vi "Calculate Curvatures.vi"(8 "error in (no error)":errorcluster, 11 "EdgeDetectionProcessor in":refnum<class "EdgeDetectionProcessor.lvclass">) -> (0 "error out":errorcluster, 3 "EdgeDetectionProcessor out":refnum<class "EdgeDetectionProcessor.lvclass">)   [LabVIEW 2018, in "EdgeDetectionProcessor.lvclass"]
uses:
  EdgeDetectionProcessor.lvclass
  C:/Program Files/National Instruments/LabVIEW 2018/user.lib/Aaron/File IO/Video/Video Processor/Video Processor.lvclass
  private/Curvature Data STYP.ctl
  2471ccb5-288c-48cc-980c-5038d1df1be7.vi
  <vilib>/Analysis/5stat.llb/RMS (DBL).vi
  <vilib>/Analysis/baseanly.llb/Mean (DBL).vi
  2471ccb5-288c-48cc-980c-5038d1df1be7.vi/1ebe9616-e55e-4f0d-8ff4-2807f1f9a203.vi
  2471ccb5-288c-48cc-980c-5038d1df1be7.vi/377cf58b-8b4d-454a-95e9-e3c545549c0f.vi
  2471ccb5-288c-48cc-980c-5038d1df1be7.vi/c9f4e0f8-7816-4916-bc5d-49cbeb604e66.vi
  2471ccb5-288c-48cc-980c-5038d1df1be7.vi/08091d57-9891-4f86-b7e8-c83c60ad9e1e.vi
  2471ccb5-288c-48cc-980c-5038d1df1be7.vi/9f18ae6c-b72e-49ca-819e-288b80c2ac08.vi
  2471ccb5-288c-48cc-980c-5038d1df1be7.vi/60678d55-dfb7-4c78-a7ca-2aeac6e8a501.vi
  <vilib>/Analysis/2dsp.llb/Derivative x(t).vi
  2471ccb5-288c-48cc-980c-5038d1df1be7.vi/1ebe9616-e55e-4f0d-8ff4-2807f1f9a203.vi/a5d5fd81-05cf-4e8b-aa3e-5fb4ea73c4ff.vi
  2471ccb5-288c-48cc-980c-5038d1df1be7.vi/377cf58b-8b4d-454a-95e9-e3c545549c0f.vi/45177a7b-6163-4512-95a4-701ed642dc24.vi
  2471ccb5-288c-48cc-980c-5038d1df1be7.vi/08091d57-9891-4f86-b7e8-c83c60ad9e1e.vi/465288f6-55f4-45e2-a969-02cddaf6938b.vi
  2471ccb5-288c-48cc-980c-5038d1df1be7.vi/9f18ae6c-b72e-49ca-819e-288b80c2ac08.vi/48fadc9c-9650-4744-b0c6-3e292434cbd4.vi
  <userlib>/Aaron/File IO/Video/Frames/Video Frame/Video Frame.lvclass
  <vilib>/Analysis/NI_AALBase.lvlib
  <vilib>/Analysis/NI_AALPro.lvlib
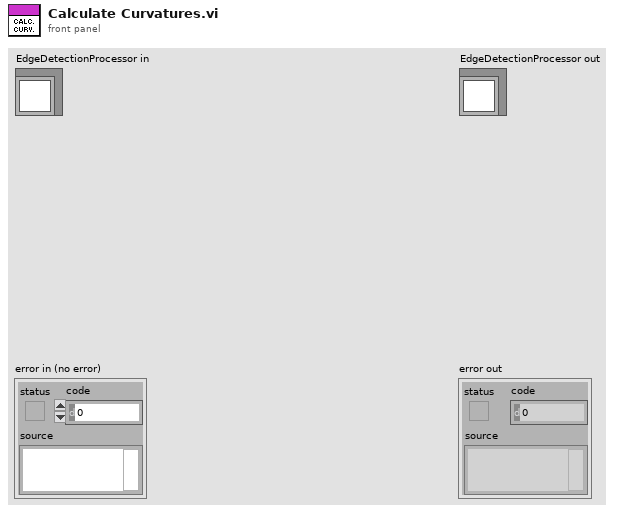
[diagram p1: front panel]
types:
  T1 = typedef "EdgeDetectionProcessor.lvclass/Curvature Data STYP.ctl" = cluster{"Discrete":dbl[], "Magnitude":dbl, "Average":dbl, "RMS":dbl}
  T2 = typedef "IMAQ ExtractCurvesCurve.ctl" = cluster{"Points":cluster{"X":dbl, "Y":dbl}[], "Closed?":bool, "Curve Length":dbl, "Min Edge Strength":dbl, "Max Edge Strength":dbl, "Average Edge Strength":dbl}
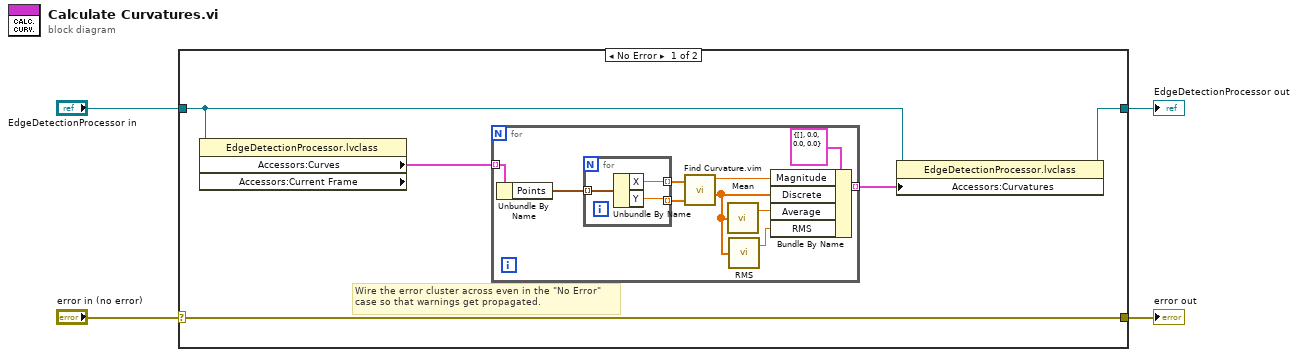
[diagram p0: block diagram]
diagram:
  n1 = case shown="No Error" "error in (no error)" {
    selector: "error in (no error)" -> [w9 w24]
    tunnel: [w9 w24] -> w3
    tunnel: [w5 w23] -> w1
    tunnel: "EdgeDetectionProcessor in" -> [w7 w23]
    frame No Error {
      # "Wire the error cluster across even in the \"No Error\"\ncase so that warnings get propagated."
      n2 = property class="EdgeDetectionProcessor.lvclass" props=["Accessors:Curves", "Accessors:Current Frame"](reference=w7) -> ("Accessors:Curves"=w8:T2[])  [unwired: 1 in, 3 out]
      n3 = for {
        tunnel: w8 -> [w19] mode=indexing
        tunnel: [w13] -> w6 mode=indexing
        n4 = Unbundle By Name(w19) -> ("Points"=w18:cluster{"X":dbl, "Y":dbl}[])
        n5 = for {
          tunnel: w18 -> [w22] mode=indexing
          tunnel: [w21] -> w17 mode=indexing
          tunnel: [w20] -> w16 mode=indexing
          n6 = Unbundle By Name(w22) -> ("X"=w21:dbl, "Y"=w20:dbl)
        }
        n7 = call "Find Curvature.vim"("Y"=w16, "X"=w17) -> ("Discrete Curvatures"=w10:dbl[], "Total Curvature"=w14:dbl)  [unwired: 8 in]
        n8 = call-poly <vilib>:"Mean.vi"("X"=w10) -> ("mean"=w12:dbl)  [unwired: 1 out]
        n9 = call-poly <vilib>:"RMS.vi"("X"=w10) -> ("rms value"=w11:dbl)  [unwired: 1 out]
        n10 = Bundle By Name(cluster=T1 {"Discrete"=[], "Magnitude"=0.0, "Average"=0.0, "RMS"=0.0} ("Curvature Data"), "Magnitude"=w14, "Discrete"=w10, "Average"=w12, "RMS"=w11) -> (w13:T1)
      }
      n11 = property class="EdgeDetectionProcessor.lvclass"(reference=w7, "Accessors:Curvatures"=w6) -> (reference out=w5:refnum<class "EdgeDetectionProcessor.lvclass">)  [unwired: 1 in, 1 out]
    }
    frame Error {
    }
  }
  "error out" <- w3
  "EdgeDetectionProcessor out" <- w1
